vi "Set Tree.vi"(8 "error in (no error)":errorcluster, 11 "[V] Sys Cfg Main in":refnum<class "[V] Sys Cfg Main.lvclass">) -> (0 "error out":errorcluster, 3 "[V] Sys Cfg Main out":refnum<class "[V] Sys Cfg Main.lvclass">)   [LabVIEW 2020, in "[V] Sys Cfg Main.lvlib" / "[V] Sys Cfg Main.lvclass"]
uses:
  [V] Sys Cfg Main.lvclass
  [V] Sys Cfg Main.lvclass/[V] Sys Cfg Main.ctl
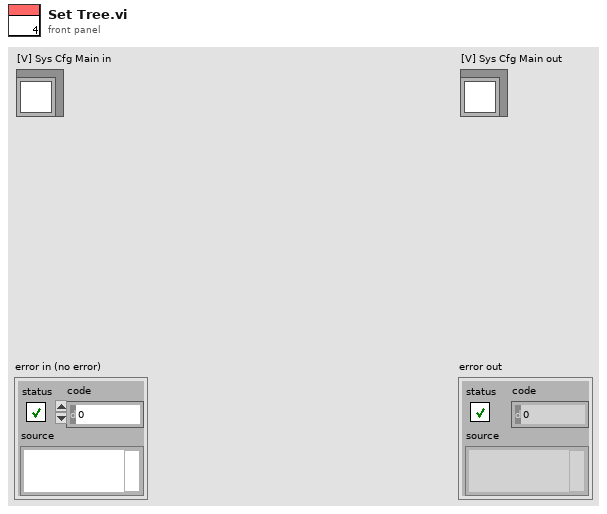
[diagram p1: front panel]
types:
  T1 = cluster{"Left Cell String":string, "Child Text":string[], "Child Tag":string, "Item Indent":i32, "Child Only?":bool, "Glyph Index":i32}
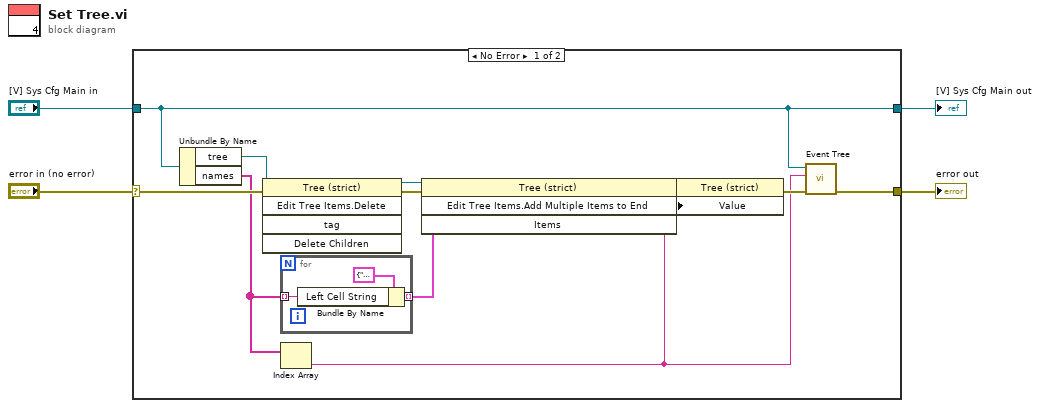
[diagram p0: block diagram]
diagram:
  n1 = case shown="No Error" "error in (no error)" {
    selector: "error in (no error)" -> [w15 w21]
    tunnel: [w5 w21] -> w3
    tunnel: [w6 w20] -> w1
    tunnel: "[V] Sys Cfg Main in" -> [w6 w20]
    frame No Error {
      n2 = Unbundle By Name(w6) -> ("tree"=w12:refnum<vi>, "names"=w9:string[])
      n3 = invoke class="Tree (strict)" method="Edit Tree Items.Delete"(reference=w12, error in=w15) -> (reference out=w13:refnum<vi>, error out=w14:errorcluster)  [unwired: 3 in, 3 out]
      n4 = for {
        tunnel: w9 -> [w18] mode=indexing
        tunnel: [w17] -> w16 mode=indexing
        n5 = Bundle By Name(cluster=T1 {"Left Cell String"="", "Child Text"=[], "Child Tag"="", "Item Indent"=0, "Child Only?"=FALSE, "Glyph Index"=0} ("Item"), "Left Cell String"=w18) -> (w17:T1)
      }
      n6 = Index Array(array=w9) -> (element=w7:string)  [unwired: 1 in]
      n7 = invoke class="Tree (strict)" method="Edit Tree Items.Add Multiple Items to End"(reference=w13, error in=w14, "Items"=w16) -> (reference out=w10:refnum<vi>, error out=w11:errorcluster)  [unwired: 1 in, 2 out]
      n8 = property class="Tree (strict)"(reference=w10, error in=w11, "Value"=w7) -> (error out=w8:errorcluster)  [unwired: 1 out]
      n9 = call "Event Tree.vi"("error in (no error)"=w8, "item"=w7, "[V] Sys Cfg Main in"=w6) -> ("error out"=w5:errorcluster)  [unwired: 7 in, 1 out]
    }
    frame Error {
    }
  }
  "error out" <- w3
  "[V] Sys Cfg Main out" <- w1
